vi "保存TDM文件.vi"() -> ()   [LabVIEW 2010]
uses:
  <vilib>/Platform/storage/lvStorage.llb/xStorage/Open Data Storage/Open Data Storage.xnode
  <vilib>/Platform/storage/lvStorage.llb/_openFunction.ctl
  <vilib>/Platform/storage/lvStorage.llb/xStorage/Write Data/Write Data.xnode
  <vilib>/Platform/storage/Storage.llb/usiOverwriteOptions.ctl
  <vilib>/Platform/storage/Storage.llb/usiSequenceRepresentation.ctl
  <vilib>/Platform/storage/lvStorage.llb/xStorage/Close Data Storage/Close Data Storage.xnode
  Instance           1 19Saved   保存TDM文件 .vi
  <vilib>/Platform/storage/lvStorage.llb/_openStorageWithRootAutoDetect.vi
  <vilib>/Platform/storage/lvStorage.llb/xStorage/xStorageSupp/ErrorOut.vi
  <vilib>/Platform/storage/Storage.llb/_createExplicitChildObject.vi
  <vilib>/Platform/storage/lvStorage.llb/_prepDDT.vi
  <vilib>/Platform/storage/lvStorage.llb/_getChannelNameFromDDT.vi
  <vilib>/Platform/storage/lvStorage.llb/_saveDDT.vi
  <vilib>/Platform/storage/Storage.llb/__savePropString.vi
  <vilib>/Platform/storage/Storage.llb/Get Object Info.vi
  <vilib>/Platform/storage/Storage.llb/__closeStorageFromObject.vi
panel:
  out "波形图":dynamicdata(graph)
  in  "文件路径":path
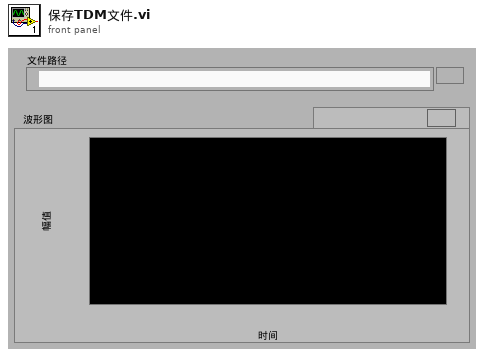
[diagram p1: front panel]
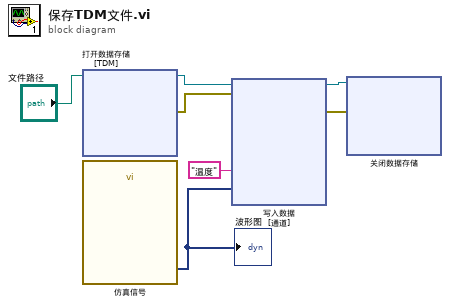
[diagram p0: block diagram]
diagram:
  n1 = xnode "打开数据存储\n[TDM]"("文件路径"="文件路径") -> ("存储引用句柄（文件）"=w7:refnum<k20>, "错误输出"=w5:errorcluster)  [unwired: 4 in, 1 out]
  n2 = call "仿真信号"() -> ("方波与均匀噪声"=w1:dynamicdata)  [unwired: 14 in, 1 out]
  "波形图" <- w1
  n3 = xnode "写入数据\n[通道]"("名称"="温度" ("传感器ID"), "信号"=w1, "存储引用句柄（文件）"=w7, "错误输入"=w5) -> ("存储引用句柄（文件） 输出"=w3:refnum<k20>, "错误输出"=w2:errorcluster)  [unwired: 2 in, 1 out]
  n4 = xnode "关闭数据存储\n"("存储引用句柄（文件）"=w3, "错误输入（无错误）"=w2) -> ()  [unwired: 2 out]
